vi "MrClean.set clean time.vi"(0 "i ref in":refnum<vi>, 2 "clean time [s]":dbl format="%.2f", 3 "ms timeout (100)":i32=100, 5 "error in (no error)":errorcluster) -> (14 "i ref out":refnum<vi>, 17 "timed out":bool, 19 "error out":errorcluster)   [LabVIEW 2014, in "MrClean.lvlib"]
doc: "Sets the time used for cleaning. This time determines the length of the Gaussian waveform produced by one of the function generators."
uses:
  MrClean.lvlib
  CSCore/CSSystem/CoreDefs/CoreDefs.error_type.ctl
  CSCore/CSSystem/CoreLib/CoreLib.double 2 byte array.vi
  CSCore/BaseProcess/BaseProcess.lvlib
  CSCore/CSSystem/CoreLib/CoreLib.lvlib
  LEBITLib/LEBITLib.lvlib
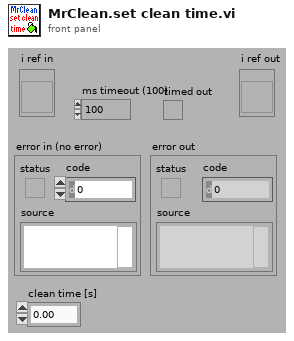
[diagram p1: front panel]
types:
  T1 = typedef "CoreDefs.error_type.ctl" = enum16{"no error", "can't load process", "can't unload process", "process does not exist", "can't install process", "can't remove process", "unknown function", "time out", "can't execute function", "duplicate queue name", "super not found", "caller queue invalid", "can't ping process", "unknown error", "VISA Error", "VISA timeout", "GPIB timeout", "GPIB error", "communication error", "data type mismatch", "can't read data from OPC server", "can't write data to OPC server", "OET error", "function not implemented", "process already exists", "invalid Shared Variable name", "error writing Shared Variable", "error reading Shared Variable", "invalid client name", "corrupt database", "unknown class", "call not authorized", "parameter out of range", "OET timeout: can't get data to modify", "invalid queue name", "requested operation incompatible with current state", "event undefined", "event disabled", "state undefined", "caller is not a friend", "EventBuilder: bad eventID", "EventBuilder: no DAQ devices", "a thread must not stop itself", "UNUSED ELEMENT4", "DiscArchiver: eventData incomplete", "DiscArchiver: eventData does not belong to run", "DiscArchiver: can't open file", "DiscArchiver: can't write to file", "DiscArchiver: available disc space low", "can't acquire semaphore", "error reading data from database", "notifier object is not existing", "can't register process", "can't unregister process", "illegal event type", "object disabled", "object already exists", "can't change state", "Instrument not found", "no connection to remote node", "invalid reference", "N/A", "UNUSED ELEMENT 1", "element not found", "illegal TCP/IP connection detected", "object does not exist", "invalid access ID", "unknown CS system", "invalid privilige", "unsupported data type", "unsupported server type", "IO server already exists", "Shared Variable already exists"}
  T2 = enum16{"simple", "synchronous", "asynchronous", "notification"}
  T3 = typedef "CoreDefs.rawDataType.ctl" = i8[]
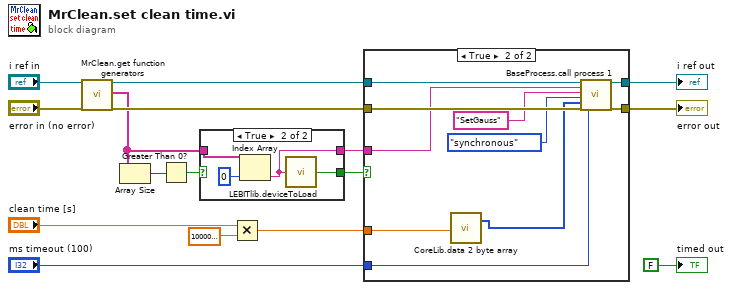
[diagram p0: block diagram]
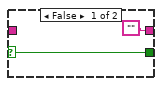
[diagram p2: hidden frame]
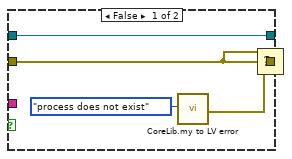
[diagram p3: hidden frame]
diagram:
  n1 = call "MrClean.get function generators.vi"("i ref in"="i ref in", "error in (no error)"="error in (no error)") -> ("i ref out"=w13:refnum<vi>, "function generators"=w4:string[], "error out"=w11:errorcluster)  [unwired: 14 in, 1 out]
  n2 = Array Size(array=w4) -> (size(s)=w14:i32)
  n3 = Greater Than 0?(x=w14) -> (x > 0?=w2:bool)
  n4 = case shown="True" w2 {
    selector: w2 -> [w18 _]
    tunnel: w4 -> [_ w21]
    tunnel: ["" w19] -> w3
    tunnel: [w18 w20] -> w1
    frame False {
    }
    frame True {
      n5 = Index Array(array=w21, index=0) -> (element=w19:string)
      n6 = call "LEBITlib.deviceToLoad.vi"("DeviceName"=w19) -> ("DeviceIsToLoad"=w20:bool)
    }
  }
  n7 = Multiply(x="clean time [s]", y=1000000.0) -> (x*y=w6:dbl)
  n8 = case shown="True" w1 {
    tunnel: w13 -> [w23 w37]
    tunnel: "ms timeout (100)" -> [_ w36]
    tunnel: w11 -> [w26 w35]
    tunnel: [w27 w34] -> w10
    tunnel: [w23 w33] -> w9
    tunnel: w6 -> [_ w29]
    tunnel: w3 -> [_ w30]
    frame False {
      n9 = call "CoreLib.my to LV error.vi"("ErrorTypes"=CoreDefs.error_type."process does not exist") -> ("myErrorCluster"=w25:errorcluster)  [unwired: 17 in, 1 out]
      n10 = Select(t=w26, s=w26, f=w25) -> (s? t:f=w27:errorcluster)
    }
    frame True {
      n11 = call-poly "CoreLib.data 2 byte array.vi"("f64"=w29) -> ("byteArray out"=w28:T3)  [unwired: 18 in]
      n12 = call "BaseProcess.call process 1.vi"("i ref in"=w37, "Object"=w30, "Selector"="SetGauss", "CallType"=T2."synchronous", "Data"=w28, "error in (no error)"=w35, "timeout (ms)"=w36) -> ("i ref out"=w33:refnum<vi>, "error out"=w34:errorcluster)  [unwired: 10 in, 1 out]
    }
  }
  "error out" <- w10
  "i ref out" <- w9
  "timed out" <- FALSE ("timed out")
